vi "startCamera.vi"(8 "error in (no error)":errorcluster, 10 "camera":string, 11 "AtomChipHWC in":refnum<class "AtomChipHWC.lvclass">) -> (0 "error out":errorcluster, 3 "AtomChipHWC out":refnum<class "AtomChipHWC.lvclass">)   [LabVIEW 2011, in "Hardware.lvlib" / "HWControllers.lvlib" / "AtomChipHWC.lvclass"]
uses:
  AtomChipHWC.lvclass
  AtomChipHWC.lvclass/AtomChipHWC.ctl
  Network Controllers/NetworkCamera/NetworkCamera.lvclass
  IntegrationManagement/CameraManager.lvclass
  Network Controllers/CameraNetworkController/CameraNetworkController.lvclass
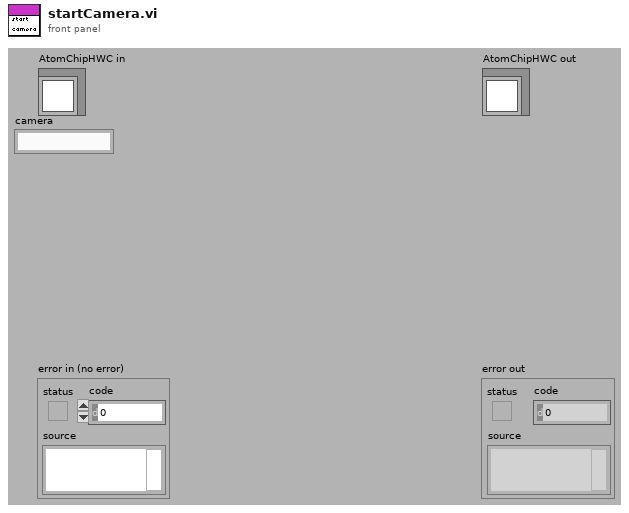
[diagram p1: front panel]
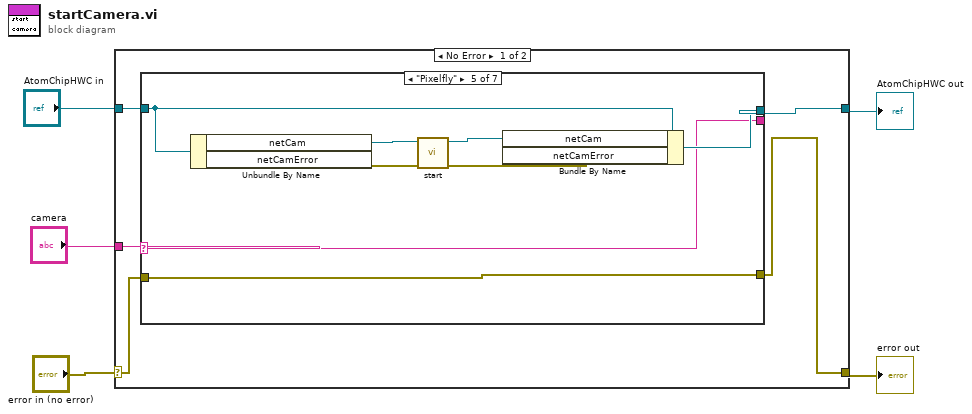
[diagram p0: block diagram]
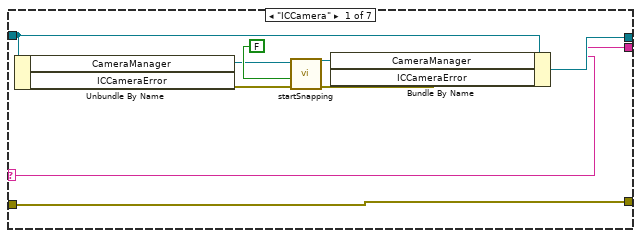
[diagram p2: hidden frame]
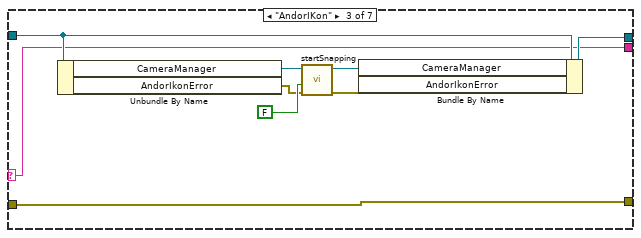
[diagram p4: hidden frame]
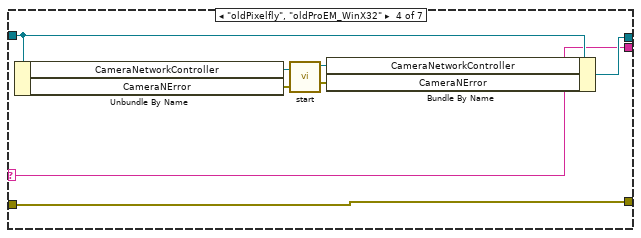
[diagram p5: hidden frame]
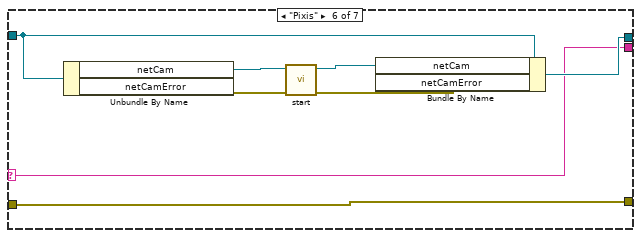
[diagram p6: hidden frame]
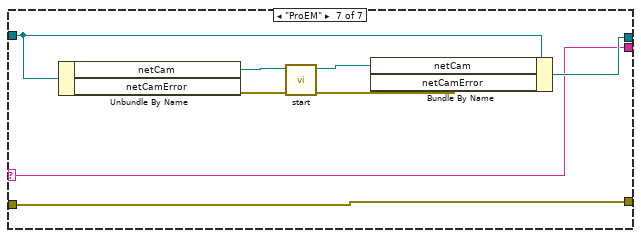
[diagram p7: hidden frame]
diagram:
  n1 = case shown="No Error" "error in (no error)" {
    selector: "error in (no error)" -> [w8 w64]
    tunnel: [w6 w64] -> w4
    tunnel: [w7 w63] -> w2
    tunnel: "AtomChipHWC in" -> [w9 w63]
    tunnel: "camera" -> [w10 _]
    frame No Error {
      n2 = case shown="\"Pixelfly\"" w10 {
        selector: w10 -> [w14 _ w25 w34 w44 w52 w60]
        tunnel: w9 -> [w15 w21 w29 w37 w46 w54 w62]
        tunnel: w8 -> [w11 w20 w22 w31 w43 w51 w59]
        tunnel: [w11 w20 w22 w31 w43 w51 w59] -> w6
        tunnel: [w16 w21 w26 w35 w45 w53 w61] -> w7
        tunnel: [w14 _ w25 w34 w44 w52 w60] -> _
        frame "ICCamera" {
          n3 = Unbundle By Name(w15) -> ("CameraManager"=w18:refnum<class "CameraManager.lvclass">, "ICCameraError"=w13:errorcluster)
          n4 = call "startSnapping.vi"("error in (no error)"=w13, "releaseWhenReady"=FALSE, "CameraManager in"=w18) -> ("error out"=w12:errorcluster, "CameraManager out"=w17:refnum<class "CameraManager.lvclass">)  [unwired: 7 in]
          n5 = Bundle By Name(cluster=w15, "CameraManager"=w17, "ICCameraError"=w12) -> (w16:refnum<class "AtomChipHWC.lvclass">)
        }
        frame Default {
        }
        frame "AndorIKon" {
          n6 = Unbundle By Name(w29) -> ("CameraManager"=w30:refnum<class "CameraManager.lvclass">, "AndorIkonError"=w24:errorcluster)
          n7 = call "startSnapping.vi"("error in (no error)"=w24, "releaseWhenReady"=FALSE, "CameraManager in"=w30) -> ("error out"=w23:errorcluster, "CameraManager out"=w28:refnum<class "CameraManager.lvclass">)  [unwired: 7 in]
          n8 = Bundle By Name(cluster=w29, "CameraManager"=w28, "AndorIkonError"=w23) -> (w26:refnum<class "AtomChipHWC.lvclass">)
        }
        frame "oldPixelfly", "oldProEM_WinX32" {
          n9 = Unbundle By Name(w37) -> ("CameraNetworkController"=w38:refnum<class "CameraNetworkController.lvclass">, "CameraNError"=w33:errorcluster)
          n10 = call "start.vi"("error in (no error)"=w33, "CameraNetworkController in"=w38) -> ("error out"=w32:errorcluster, "CameraNetworkController out"=w36:refnum<class "CameraNetworkController.lvclass">)  [unwired: 8 in]
          n11 = Bundle By Name(cluster=w37, "CameraNetworkController"=w36, "CameraNError"=w32) -> (w35:refnum<class "AtomChipHWC.lvclass">)
        }
        frame "Pixelfly" {
          n12 = Unbundle By Name(w46) -> ("netCam"=w42:refnum<class "NetworkCamera.lvclass">, "netCamError"=w40:errorcluster)
          n13 = call-dynamic "start.vi"("error in (no error)"=w40, "NetworkCamera in"=w42) -> ("error out"=w39:errorcluster, "NetworkCamera out"=w41:refnum<class "NetworkCamera.lvclass">)  [unwired: 8 in]
          n14 = Bundle By Name(cluster=w46, "netCam"=w41, "netCamError"=w39) -> (w45:refnum<class "AtomChipHWC.lvclass">)
        }
        frame "Pixis" {
          n15 = Unbundle By Name(w54) -> ("netCam"=w50:refnum<class "NetworkCamera.lvclass">, "netCamError"=w48:errorcluster)
          n16 = call-dynamic "start.vi"("error in (no error)"=w48, "NetworkCamera in"=w50) -> ("error out"=w47:errorcluster, "NetworkCamera out"=w49:refnum<class "NetworkCamera.lvclass">)  [unwired: 8 in]
          n17 = Bundle By Name(cluster=w54, "netCam"=w49, "netCamError"=w47) -> (w53:refnum<class "AtomChipHWC.lvclass">)
        }
        frame "ProEM" {
          n18 = Unbundle By Name(w62) -> ("netCam"=w58:refnum<class "NetworkCamera.lvclass">, "netCamError"=w56:errorcluster)
          n19 = call-dynamic "start.vi"("error in (no error)"=w56, "NetworkCamera in"=w58) -> ("error out"=w55:errorcluster, "NetworkCamera out"=w57:refnum<class "NetworkCamera.lvclass">)  [unwired: 8 in]
          n20 = Bundle By Name(cluster=w62, "netCam"=w57, "netCamError"=w55) -> (w61:refnum<class "AtomChipHWC.lvclass">)
        }
      }
    }
    frame Error {
    }
  }
  "error out" <- w4
  "AtomChipHWC out" <- w2
